vi "PlugandPlayPmod.vi"() -> ()   [LabVIEW 2014]
uses:
  <vilib>/MakerHub/LINX/Public/Sensors/Accelerometer/ADXL345/Address.ctl
  <vilib>/MakerHub/LINX/LMH-LINX.lvlib
  <vilib>/MakerHub/LINX/Public/Sensors/Accelerometer/ADXL345/ADXL345.lvlib
panel:
  in  "I2C Channel (0)":u8
  in  "CS Channel":u8=10
  in  "SPI Channel (0)":u8
  in  "Serial Port":refnum<visa-resource-name>="N/A"
  in  "SPI or I2C":enum32{"SPI", "I2C"}(tab)
  in  "SPI Pmod":T1(tab)
  out "Light Level (%)":dbl
  in  "Stop Button 5":bool
  in  "LEDs":enum16{"None", "LD1", "LD2", "Both"}(ring)
  out "Buttons":u8
  out "X - Axis":string
  out "Y - Axis":string
  in  "Stop Button 6":bool
  in  "Supply Voltage":dbl=3.3
  out "PmodMIC3":dbl(graph)
  in  "Stop Button 7":bool
  out "Voltage (V)":dbl
  out "PmodTC1":T2(graph)
  out "Temperatures":T3
  in  "Stop Button 8":bool
  in  "I2C Pmod":T4(tab)
  out "Acceleration Data (g)":T5
  in  "Stop Button":bool
  in  "ADXL345 Address":T6
  in  "Resolution (g)":enum16{"2g", "4g", "8g", "16g"}(ring)
  out "PmodACL":T5(graph)
  out "PmodCMPS":T7(graph)
  out "Gauss":cluster{"X":dbl, "Y":dbl, "Z":dbl}
  in  "Stop Button 2":bool
  in  "Address":enum8{"0x68", "0x69"}(ring)=enum."0x69"
  in  "Resolution (dps)":enum16{"2000", "500", "250"}(ring)
  out "PmodGYRO":cluster{"X":i16, "Y":i16, "Z":i16}(graph)
  in  "Stop Button 3":bool
  out "Gyro XYZ (degrees/sec)":cluster{"X":i16, "Y":i16, "Z":i16}
  out "PmodTMP3":dbl(graph)
  out "Ambient Temperature (C)":dbl
  in  "Slave Address":T8(ring)
  in  "Resolution":enum16{"0.5", "0.25", "0.125", "0.0625"}(ring)
  in  "Stop Button 4":bool
  # "LINX Setup"
  # "Choose SPI or I2C and Choose the Pmod You Are Using"
  # "PmodALS\n\nThis example demonstrates how to read the relative light sensed by the PmodALS.\n\nInstructions:\n1. Click the Run Arrow."
  # "PmodJSTK\n\nThis example demonstrates how to read XY data, button pushes, and set LEDs on the PmodJSTK.\n\nInstructions:\n1. Select the LEDs you want on.\n2. Click the Run Arrow."
  # "PmodJSTK Button Layout"
  # "Joystick Button = Bit 1\nButton 1 = Bit 2\nButton 2 = Bit 3"
  # "Combinations"
  # "Bit 3 | Bit 2 | Bit 1"
  # "Result"
  # "0        0         0\n0        0         1\n0        1         0\n0        1         1\n1        0         0\n1        0         1\n1        1         0\n1        1         1"
  # "0\n1\n2\n3\n4\n5\n6\n7"
  # "PmodMIC3\n\nThis example demonstrates how to read the voltage values from the PmodMIC3.\n\nInstructions:\n1. Enter the Supply Voltage used.\n2. Click the Run Arrow."
  # "PmodTC1\n\nThis example demonstrates how to read the thermocouple and reference temperatures from the PmodTC1.\n\nInstructions:\n1. Click the Run Arrow."
  # "PmodACL\n\nThis example demonstrates how to read the acceleration sensed by the PmodACL.\n\nInstructions:\n1. Select the Address (default 0x1D)\n2. Select the desired resolution (2g, 4g, 8g, 16g)\n3. Click the Run Arrow."
  # "PmodCMPS\n\nThis example demonstrates how to read the angular velocity values from the CMPS.\n\nInstructions:\n1. Click the Run Arrow."
  # "PmodGYRO\n\nThis example demonstrates how to read the angular velocity values from the PmodGYRO.\n\nInstructions:\n1. Select the Slave Address for the Pmod (default 0x69)\n2. Select the desired resolution.\n3. Click the Run Arrow."
  # "PmodTMP3\n\nThis example demonstrates how to read the angular velocity values from the PmodTMP3.\n\nInstructions:\n1. Select the Slave Address for the Pmod (default 0x48 with all jumpers to ground)\n2. Select the desired resolution.\n3. Click the Run Arrow."
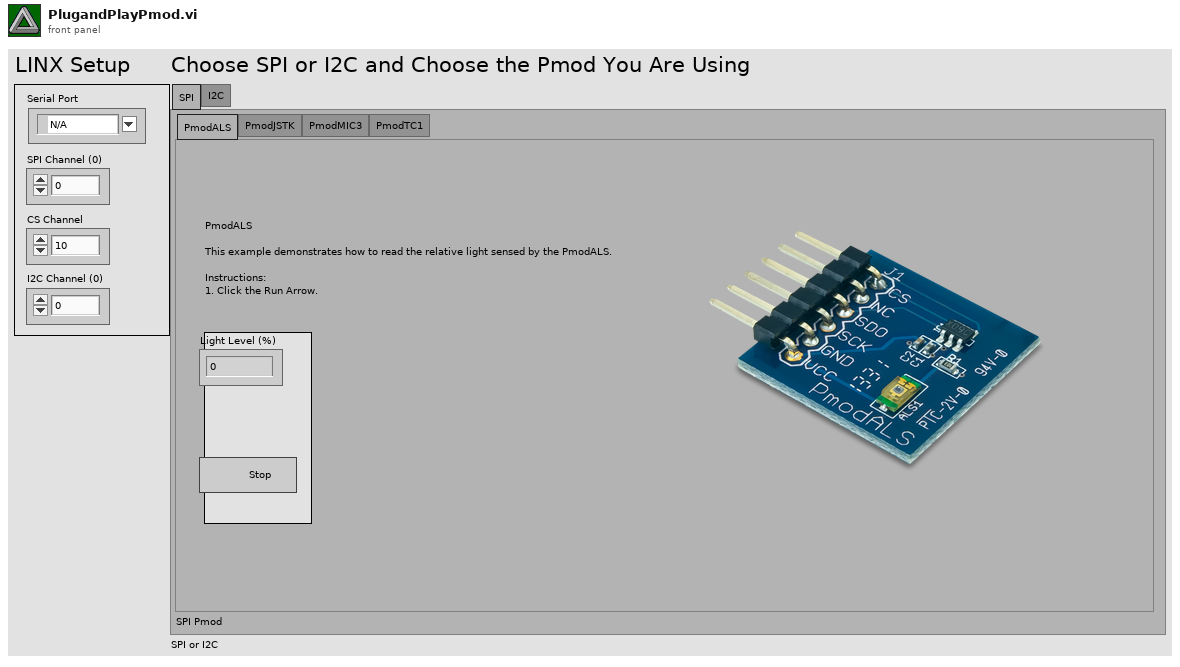
[diagram p1: front panel]
types:
  T1 = enum32{"PmodALS", "PmodJSTK", "PmodMIC3", "PmodTC1"}
  T2 = cluster{"Cold Junction (C)":i16, "Thermocouple (C)":i16}
  T3 = cluster{"Thermocouple (C)":i16, "Cold Junction/Reference (C)":i16}
  T4 = enum32{"PmodACL", "PmodCMPS", "PmodGYRO", "PmodTMP3"}
  T5 = cluster{"X Axis":dbl, "Y Axis":dbl, "Z Axis":dbl}
  T6 = typedef "LMH-LINX.lvlib/ADXL345.lvlib/Address.ctl" = enum16{"0x1D (ALT High)", "0x53 (ALT Low)"}
  T7 = cluster{"Decimal I16":dbl, "Decimal I16":dbl, "Decimal I16":dbl}
  T8 = enum8{"0x48", "0x49", "0x4A", "0x4B", "0x4C", "0x4D", "0x4E", "0x4F"}
  T9 = typedef "LMH-LINX.lvlib/LINX Ref.ctl" = cluster{"Platform":T10, "Interface":T11, "LINX Device Config":T12}
  T10 = typedef "LMH-LINX.lvlib/Platform.ctl" = enum16{"LINX", "myRIO"}
  T11 = typedef "LMH-LINX.lvlib/Interface.ctl" = enum16{"Serial", "TCP"}
  T12 = typedef "LMH-LINX.lvlib/Device.lvlib/LINX Device Config.ctl" = cluster{"Interface":T11, "COM Port":refnum<visa-resource-name>, "TCP Configuration":T13, "Device Family":u8, "Device ID":u8, "Device Name":string, "TCP Ref":refnum<k5>, "Channels":T14}
  T13 = typedef "LMH-LINX.lvlib/Device.lvlib/TCP Config.ctl" = cluster{"IP Address":string, "Port":u16}
  T14 = typedef "LMH-LINX.lvlib/Channels.ctl" = cluster{"DI":u8[], "DO":u8[], "AI":u8[], "AO":u8[], "PWM":u8[], "QE":u8[], "UART":u8[], "I2C 2":u8[], "SPI":u8[], "CAN":u8[], "Servo":u8[], "AI Ref (V)":dbl, "AO Ref (V)":dbl, "AO Resolution (Bits)":u8}
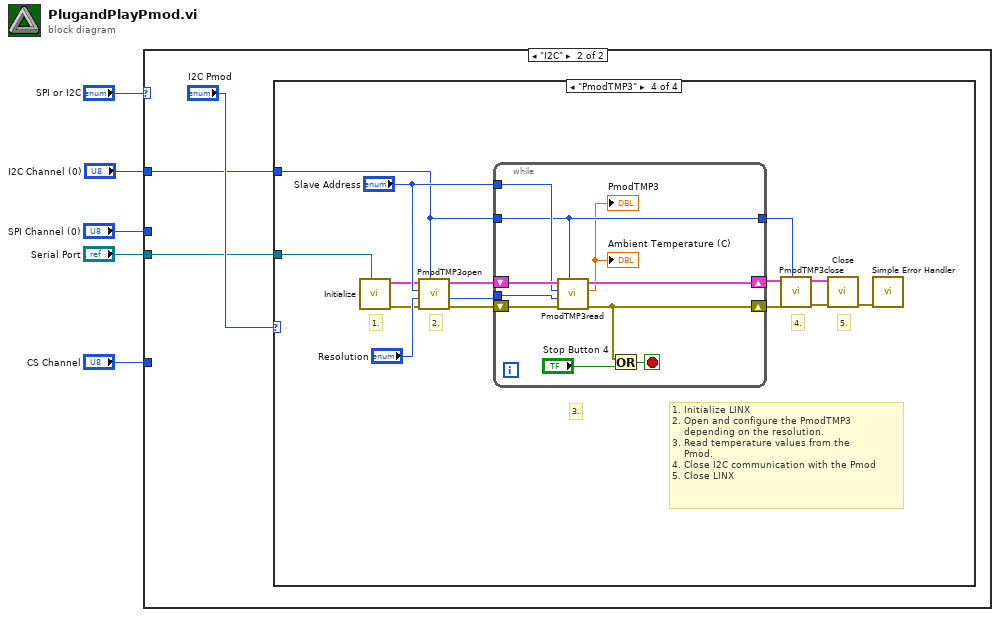
[diagram p0: block diagram]
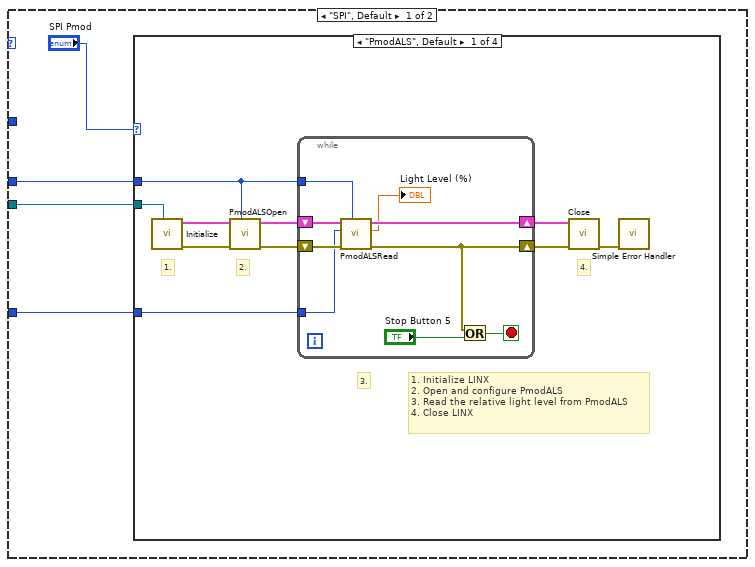
[diagram p2: hidden frame]
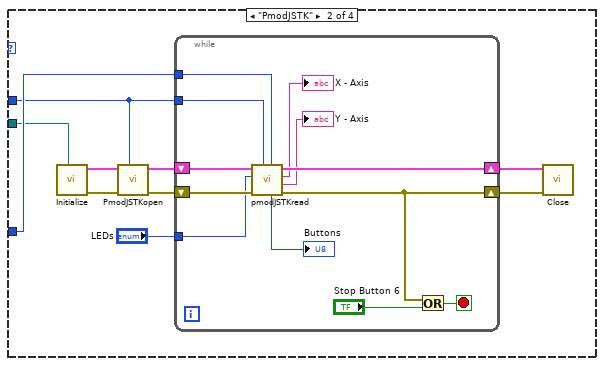
[diagram p3: hidden frame]
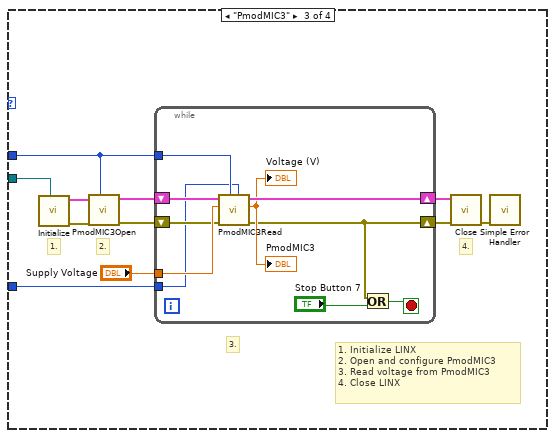
[diagram p4: hidden frame]
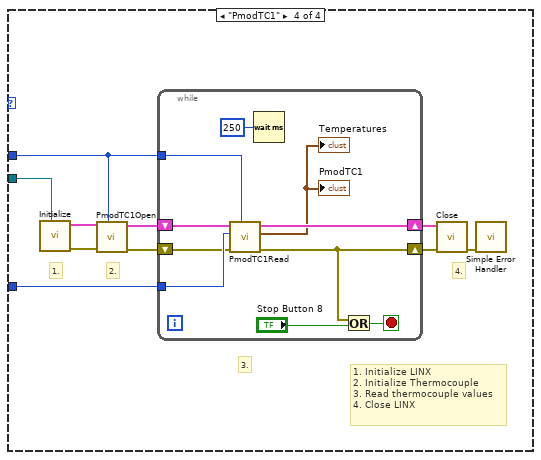
[diagram p5: hidden frame]
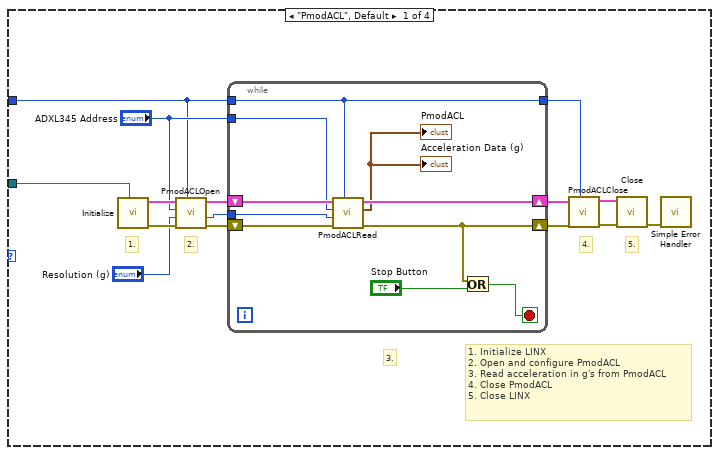
[diagram p6: hidden frame]
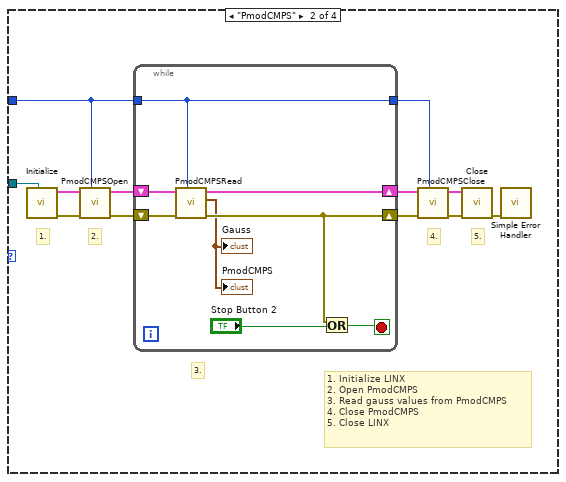
[diagram p7: hidden frame]
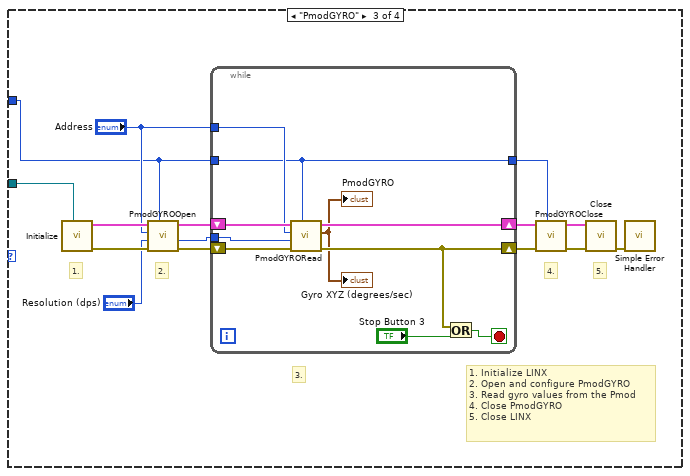
[diagram p8: hidden frame]
diagram:
  n1 = case shown="\"I2C\"" "SPI or I2C" {
    tunnel: "Serial Port" -> [w8 w92]
    tunnel: "CS Channel" -> [w7 _]
    tunnel: "SPI Channel (0)" -> [w6 _]
    tunnel: "I2C Channel (0)" -> [_ w93]
    frame "SPI", Default {
      n2 = case shown="\"PmodALS\", Default" "SPI Pmod" {
        tunnel: w8 -> [w15 w29 w52 w74]
        tunnel: w7 -> [w16 w31 w51 w73]
        tunnel: w6 -> [w12 w30 w53 w72]
        frame "PmodALS", Default {
          # "4."
          # "3."
          # "1. Initialize LINX\n2. Open and configure PmodALS\n3. Read the relative light level from PmodALS\n4. Close LINX"
          # "2."
          # "1."
          n3 = call <vilib>:"Initialize.vi"("Serial Port"=w15) -> ("Error Out"=w13:errorcluster, "LINX Ref"=w14:T9)  [unwired: 8 in, 1 out]
          n4 = call "PmodALSOpen.vi"("SPI Channel (0)"=w12, "error in (no error)"=w13, "LINX Ref"=w14) -> ("error out"=w10:errorcluster, "LINX Resource"=w11:T9)  [unwired: 6 in, 1 out]
          n5 = while {
            shift-right: [w24] -> w18
            shift-left: w11 -> [w26]
            shift-right: [w20] -> w19
            shift-left: w10 -> [w25]
            tunnel: w16 -> [w21]
            tunnel: w12 -> [w22]
            stop <- w28 stop-if-true
            n6 = call "PmodALSRead.vi"("SPI Channel (0)"=w22, "error in (no error)"=w25, "CS Channel"=w21, "LINX Resource in"=w26) -> ("error out"=w20:errorcluster, "Light Level (%)"=→"Light Level (%)":dbl, "LINX Resource out"=w24:T9)  [unwired: 5 in]
            n7 = Or(x=w20, y="Stop Button 5") -> (x .or. y?=w28:bool)
          }
          n8 = call <vilib>:"Close.vi"("Error In"=w19, "LINX Resource"=w18) -> ("Error Out"=w17:errorcluster)  [unwired: 8 in, 1 out]
          n9 = call <vilib>:"Simple Error Handler.vi"("error in (no error)"=w17) -> ()  [unwired: 4 in, 5 out]
        }
        frame "PmodJSTK" {
          n10 = call <vilib>:"Initialize.vi"("Serial Port"=w29) -> ("Error Out"=w33:errorcluster, "LINX Ref"=w32:T9)  [unwired: 8 in, 1 out]
          n11 = call "PmodJSTKopen.vi"("SPI Channel (0)"=w30, "error in (no error)"=w33, "LINX Ref"=w32) -> ("error out"=w35:errorcluster, "LINX Resource"=w34:T9)  [unwired: 7 in]
          n12 = while {
            tunnel: w30 -> [w43]
            tunnel: w31 -> [w41]
            shift-right: [w49] -> w36
            shift-left: w34 -> [w44]
            shift-right: [w47] -> w37
            shift-left: w35 -> [w50]
            tunnel: "LEDs" -> [w39]
            stop <- w48 stop-if-true
            n13 = call "pmodJSTKread.vi"("CS Channel"=w41, "SPI Channel (0)"=w43, "error in (no error)"=w50, "LEDs"=w39, "LINX Resource in"=w44) -> ("error out"=w47:errorcluster, "Y - Axis"=→"Y - Axis":string, "X - Axis"=→"X - Axis":string, "LINX Resource out"=w49:T9, "Buttons"=→"Buttons":u8)  [unwired: 2 in]
            n14 = Or(x=w47, y="Stop Button 6") -> (x .or. y?=w48:bool)
          }
          n15 = call <vilib>:"Close.vi"("Error In"=w37, "LINX Resource"=w36) -> ()  [unwired: 8 in, 2 out]
        }
        frame "PmodMIC3" {
          # "1. Initialize LINX\n2. Open and configure PmodMIC3\n3. Read voltage from PmodMIC3\n4. Close LINX"
          # "4."
          # "3."
          # "2."
          # "1."
          n16 = call <vilib>:"Initialize.vi"("Serial Port"=w52) -> ("Error Out"=w57:errorcluster, "LINX Ref"=w58:T9)  [unwired: 8 in, 1 out]
          n17 = call "PmodMIC3Open.vi"("SPI Channel (0)"=w53, "error in (no error)"=w57, "LINX Ref"=w58) -> ("error out"=w56:errorcluster, "LINX Resource"=w55:T9)  [unwired: 6 in, 1 out]
          n18 = while {
            tunnel: "Supply Voltage" -> [w71]
            tunnel: w53 -> [w70]
            shift-right: [w64] -> w59
            shift-left: w56 -> [w68]
            shift-right: [w67] -> w60
            shift-left: w55 -> [w69]
            tunnel: w51 -> [w62]
            stop <- w65 stop-if-true
            n19 = call "PmodMIC3Read.vi"("CS Channel"=w62, "SPI Channel (0)"=w70, "error in (no error)"=w68, "Supply Voltage"=w71, "LINX Resource in"=w69) -> ("error out"=w64:errorcluster, "Voltage (V)"=→"Voltage (V)" →"PmodMIC3":dbl, "LINX Resource out"=w67:T9)  [unwired: 4 in]
            n20 = Or(x=w64, y="Stop Button 7") -> (x .or. y?=w65:bool)
          }
          n21 = call <vilib>:"Close.vi"("Error In"=w59, "LINX Resource"=w60) -> ("Error Out"=w61:errorcluster)  [unwired: 8 in, 1 out]
          n22 = call <vilib>:"Simple Error Handler.vi"("error in (no error)"=w61) -> ()  [unwired: 4 in, 5 out]
        }
        frame "PmodTC1" {
          # "1. Initialize LINX\n2. Initialize Thermocouple\n3. Read thermocouple values\n4. Close LINX"
          # "4."
          # "3."
          # "2."
          # "1."
          n23 = call <vilib>:"Initialize.vi"("Serial Port"=w74) -> ("Error Out"=w77:errorcluster, "LINX Ref"=w76:T9)  [unwired: 8 in, 1 out]
          n24 = call "PmodTC1Open.vi"("SPI Channel (0)"=w72, "error in (no error)"=w77, "LINX Ref"=w76) -> ("error out"=w79:errorcluster, "LINX Resource"=w78:T9)  [unwired: 6 in, 1 out]
          n25 = while {
            tunnel: w73 -> [w91]
            tunnel: w72 -> [w90]
            shift-right: [w87] -> w80
            shift-left: w78 -> [w89]
            shift-right: [w86] -> w81
            shift-left: w79 -> [w88]
            stop <- w85 stop-if-true
            n26 = call "PmodTC1Read.vi"("SPI Channel (0)"=w90, "error in (no error)"=w88, "CS Channel"=w91, "LINX Resource in"=w89) -> ("error out"=w86:errorcluster, "Temperatures"=→"Temperatures" →"PmodTC1":T2, "LINX Resource out"=w87:T9)  [unwired: 5 in]
            n27 = Wait (ms)(milliseconds to wait=u32 250) -> ()  [unwired: 1 out]
            n28 = Or(x=w86, y="Stop Button 8") -> (x .or. y?=w85:bool)
          }
          n29 = call <vilib>:"Close.vi"("Error In"=w81, "LINX Resource"=w80) -> ("Error Out"=w75:errorcluster)  [unwired: 8 in, 1 out]
          n30 = call <vilib>:"Simple Error Handler.vi"("error in (no error)"=w75) -> ()  [unwired: 4 in, 5 out]
        }
      }
    }
    frame "I2C" {
      n31 = case shown="\"PmodTMP3\"" "I2C Pmod" {
        tunnel: w93 -> [w97 w121 w141 w166]
        tunnel: w92 -> [w108 w120 w140 w165]
        frame "PmodACL", Default {
          # "1. Initialize LINX\n2. Open and configure PmodACL\n3. Read acceleration in g's from PmodACL\n4. Close PmodACL\n5. Close LINX"
          # "5."
          # "4."
          # "3."
          # "2."
          # "1."
          n32 = call <vilib>:"Initialize.vi"("Serial Port"=w108) -> ("Error Out"=w106:errorcluster, "LINX Ref"=w107:T9)  [unwired: 8 in, 1 out]
          n33 = call "PmodACLOpen.vi"("I2C Channel (0)"=w97, "Error In"=w106, "Resolution"="Resolution (g)", "ADXL345 Address"="ADXL345 Address", "LINX Resource"=w107) -> ("Error Out"=w105:errorcluster, "Resolution"=w96:enum16{"2g", "4g", "8g", "16g"}, "LINX Resource"=w104:T9)  [unwired: 4 in]
          n34 = while {
            tunnel: "ADXL345 Address" -> [w112]
            shift-right: [w115] -> w103
            shift-left: w104 -> [w117]
            shift-right: [w110] -> w102
            shift-left: w105 -> [w116]
            tunnel: w97 -> [w111]
            tunnel: w96 -> [w113]
            tunnel: [w111] -> w95
            stop <- w118 stop-if-true
            n35 = call "PmodACLRead.vi"("I2C Channel (0)"=w111, "Error In"=w116, "Resolution"=w113, "ADXL345 Address"=w112, "LINX Resource"=w117) -> ("Error Out"=w110:errorcluster, "Acceleration Data (g)"=→"Acceleration Data (g)" →"PmodACL":T5, "LINX Resource"=w115:T9)  [unwired: 4 in]
            n36 = Or(x=w110, y="Stop Button") -> (x .or. y?=w118:bool)
          }
          n37 = call "PmodACLClose.vi"("I2C Channel (0)"=w95, "Error In"=w102, "LINX Resource"=w103) -> ("Error Out"=w100:errorcluster, "LINX Resource"=w101:T9)  [unwired: 7 in]
          n38 = call <vilib>:"Close.vi"("Error In"=w100, "LINX Resource"=w101) -> ("Error Out"=w109:errorcluster)  [unwired: 8 in, 1 out]
          n39 = call <vilib>:"Simple Error Handler.vi"("error in (no error)"=w109) -> ()  [unwired: 4 in, 5 out]
        }
        frame "PmodCMPS" {
          # "1. Initialize LINX\n2. Open PmodCMPS\n3. Read gauss values from PmodCMPS\n4. Close PmodCMPS\n5. Close LINX"
          # "5."
          # "4."
          # "3."
          # "2."
          # "1."
          n40 = call <vilib>:"Initialize.vi"("Serial Port"=w120) -> ("Error Out"=w130:errorcluster, "LINX Ref"=w131:T9)  [unwired: 8 in, 1 out]
          n41 = call "PmodCMPSOpen.vi"("I2C Channel (0)"=w121, "error in (no error)"=w130, "LINX Ref"=w131) -> ("error out"=w124:errorcluster, "LINX Resource"=w125:T9)  [unwired: 7 in]
          n42 = while {
            shift-right: [w136] -> w122
            shift-left: w125 -> [w133]
            shift-right: [w135] -> w128
            shift-left: w124 -> [w139]
            tunnel: w121 -> [w132]
            tunnel: [w132] -> w123
            stop <- w137 stop-if-true
            n43 = call "PmodCMPSRead.vi"("I2C Channel (0)"=w132, "error in (no error)"=w139, "LINX Resource in"=w133) -> ("error out"=w135:errorcluster, "Compass (Gauss)"=→"Gauss" →"PmodCMPS":cluster{"X":dbl, "Y":dbl, "Z":dbl}, "LINX Resource out"=w136:T9)  [unwired: 6 in]
            n44 = Or(x=w135, y="Stop Button 2") -> (x .or. y?=w137:bool)
          }
          n45 = call "PmodCMPSClose.vi"("I2C Channel (0)"=w123, "error in (no error)"=w128, "LINX Resource in"=w122) -> ("error out"=w126:errorcluster, "LINX Resource out"=w127:T9)  [unwired: 7 in]
          n46 = call <vilib>:"Close.vi"("Error In"=w126, "LINX Resource"=w127) -> ("Error Out"=w129:errorcluster)  [unwired: 8 in, 1 out]
          n47 = call <vilib>:"Simple Error Handler.vi"("error in (no error)"=w129) -> ()  [unwired: 4 in, 5 out]
        }
        frame "PmodGYRO" {
          # "1. Initialize LINX\n2. Open and configure PmodGYRO\n3. Read gyro values from the Pmod\n4. Close PmodGYRO\n5. Close LINX"
          # "3."
          # "5."
          # "4."
          # "2."
          # "1."
          n48 = call <vilib>:"Initialize.vi"("Serial Port"=w140) -> ("Error Out"=w150:errorcluster, "LINX Ref"=w151:T9)  [unwired: 8 in, 1 out]
          n49 = call "PmodGYROOpen.vi"("I2C Channel (0)"=w141, "error in (no error)"=w150, "Resolution (dps)"="Resolution (dps)", "Address"="Address", "LINX Ref"=w151) -> ("error out"=w147:errorcluster, "Resolution (dps)"=w144:enum16{"2000", "500", "250"}, "LINX Resource"=w149:T9)  [unwired: 4 in]
          n50 = while {
            shift-right: [w163] -> w148
            shift-left: w149 -> [w164]
            shift-right: [w158] -> w146
            shift-left: w147 -> [w162]
            tunnel: w144 -> [w161]
            tunnel: "Address" -> [w160]
            tunnel: w141 -> [w159]
            tunnel: [w159] -> w142
            stop <- w156 stop-if-true
            n51 = call "PmodGYRORead.vi"("I2C Channel (0)"=w159, "error in (no error)"=w162, "Resolution (dps)"=w161, "Address"=w160, "LINX Resource in"=w164) -> ("error out"=w158:errorcluster, "Gyro XYZ (degrees/sec)"=→"Gyro XYZ (degrees/sec)" →"PmodGYRO":cluster{"X":i16, "Y":i16, "Z":i16}, "LINX Resource out"=w163:T9)  [unwired: 4 in]
            n52 = Or(x=w158, y="Stop Button 3") -> (x .or. y?=w156:bool)
          }
          n53 = call "PmodGYROClose.vi"("I2C Channel (0)"=w142, "error in (no error)"=w146, "LINX Resource in"=w148) -> ("error out"=w153:errorcluster, "LINX Resource out"=w152:T9)  [unwired: 7 in]
          n54 = call <vilib>:"Close.vi"("Error In"=w153, "LINX Resource"=w152) -> ("Error Out"=w154:errorcluster)  [unwired: 8 in, 1 out]
          n55 = call <vilib>:"Simple Error Handler.vi"("error in (no error)"=w154) -> ()  [unwired: 4 in, 5 out]
        }
        frame "PmodTMP3" {
          # "1. Initialize LINX\n2. Open and configure the PmodTMP3\n    depending on the resolution.\n3. Read temperature values from the\n    Pmod.\n4. Close I2C communication with the Pmod\n5. Close LINX"
          # "3."
          # "5."
          # "4."
          # "2."
          # "1."
          n56 = call <vilib>:"Initialize.vi"("Serial Port"=w165) -> ("Error Out"=w168:errorcluster, "LINX Ref"=w167:T9)  [unwired: 8 in, 1 out]
          n57 = call "PmodTMP3open.vi"("I2C Channel (0)"=w166, "error in (no error)"=w168, "Resolution"="Resolution", "Slave Address"="Slave Address", "LINX Ref"=w167) -> ("error out"=w174:errorcluster, "Resolution"=w177:enum16{"0.5", "0.25", "0.125", "0.0625"}, "LINX Resource"=w173:T9)  [unwired: 4 in]
          n58 = while {
            tunnel: "Slave Address" -> [w182]
            tunnel: w166 -> [w181]
            shift-right: [w189] -> w179
            shift-left: w173 -> [w183]
            shift-right: [w185] -> w169
            shift-left: w174 -> [w188]
            tunnel: [w181] -> w178
            tunnel: w177 -> [w184]
            stop <- w187 stop-if-true
            n59 = call "PmodTMP3read.vi"("I2C Channel (0)"=w181, "error in (no error)"=w188, "Resolution"=w184, "Slave Address"=w182, "LINX Resource in"=w183) -> ("error out"=w185:errorcluster, "Ambient Temperature (C)"=→"Ambient Temperature (C)" →"PmodTMP3":dbl, "LINX Resource out"=w189:T9)  [unwired: 4 in]
            n60 = Or(x=w185, y="Stop Button 4") -> (x .or. y?=w187:bool)
          }
          n61 = call "PmodTMP3close.vi"("I2C Channel (0)"=w178, "error in (no error)"=w169, "LINX Resource in"=w179) -> ("error out"=w170:errorcluster, "LINX Resource out"=w171:T9)  [unwired: 7 in]
          n62 = call <vilib>:"Close.vi"("Error In"=w170, "LINX Resource"=w171) -> ("Error Out"=w172:errorcluster)  [unwired: 8 in, 1 out]
          n63 = call <vilib>:"Simple Error Handler.vi"("error in (no error)"=w172) -> ()  [unwired: 4 in, 5 out]
        }
      }
    }
  }
